vi "water-archive.vi"(1 "C1NI6071E":T1 {"63 ACH63 b100 Libre ?" format="%.3f"; "62 ACH62 b98 Libre ?" format="%.3f"; "61 ACH61 b96 Libre ?" format="%.3f"; "60 ACH60 b94 Libre ?" format="%.3f"; "59 ACH59 b92 Libre ?" format="%.3f"; "58 ACH58 b90 Libre ?" format="%.3f"; "57 ACH57 b88 Libre ?" format="%.3f"; "56 ACH56 b86 Libre ?" format="%.3f"; "55 ACH55 b99 Libre ?" format="%.3f"; "54 ACH54 b97 Libre ?" format="%.3f"; "53 ACH53 b95 Libre ?" format="%.3f"; "52 ACH52 b93 Libre ?" format="%.3f"; "51 ACH51 b91 Libre ?" format="%.3f"; "50 ACH50 b89 Libre ?" format="%.3f"; "49 ACH49 b87 Libre ?" format="%.3f"; "48 ACH48 b85 Réservé" format="%.3f"; "47 ACH47 b84 Réservé" format="%.3f"; "46 ACH46 b82 Réservé" format="%.3f"; "45 ACH45 b80 Mesure phase HF1" format="%.3f"; "44 ACH44 b78 Mesure Atténuateur" format="%.3f"; "43 ACH43 b74 Réservé" format="%.3f"; "42 ACH42 b72 Mes champ Dipôle 2" format="%.3f"; "41 ACH41 b70 Mes H5" format="%.3f"; "40 ACH40 b68 Mes I correcte Dipôle 21 (H4)" format="%.3f"; "39 ACH39 b83 Réservé" format="%.3f"; "38 ACH38 b81 Mesure phase HF2" format="%.3f"; "37 ACH37 b79 Mes position Déphaseur ajust" format="%.3f"; "36 ACH36 b77 Mes position Déphaseur" format="%.3f"; "35 ACH35 b73 Mes champ Dipôle 2" format="%.3f"; "34 ACH34 b71 Mes I Guidage V5" format="%.3f"; "33 ACH33 b69 Mes I Guidage V4" format="%.3f"; "32 ACH32 b67 Mes I Guidage V3" format="%.3f"; "31 ACH31 b66 Mes I correcte Dipôle 1 (H3)" format="%.3f"; "30 ACH30 b64 Mes I Guidage H2" format="%.3f"; "29 ACH29 b62 Mes I Guidage H1" format="%.3f"; "28 ACH28 b60 Mes I Dipôle 1" format="%.3f"; "27 ACH27 b58 Mes I Quadripôle 2" format="%.3f"; "26 ACH26 b56 Réservé" format="%.3f"; "25 ACH25 b54 Mes I Triplet 2-1" format="%.3f"; "24 ACH24 b52 Mes I Triplet 1-2" format="%.3f"; "23 ACH23 b65 Mes I Guidage V2" format="%.3f"; "22 ACH22 b63 Mes I Guidage V1" format="%.3f"; "21 ACH21 b61 Mes I Dipôle 2" format="%.3f"; "20 ACH20 b59 Mes I Solénoïde" format="%.3f"; "19 ACH19 b57 Mes I Quadripôle 1" format="%.3f"; "18 ACH18 b55 Mes I Triplet 2-2" format="%.3f"; "17 ACH17 b53 Réservé" format="%.3f"; "16 ACH16 b51 Mes I Triplet 1-1" format="%.3f"; "15 ACH15 b18 Libre ?" format="%.3f"; "14 ACH14 b16 Libre ?" format="%.3f"; "13 ACH13 b14 Libre ?" format="%.3f"; "12 ACH12 b12 Mes Vide jauge canon" format="%.3f"; "11 ACH11 b10 Mes Vide DIP 1 (PIQ27 + 33)" format="%.3f"; "10 ACH10 b08 Mes Vide Section (PIQ 16)" format="%.3f"; "09 ACH09 b06 Mes Vide SAS guide HF" format="%.3f"; "08 ACH08 b04 Mes température Section" format="%.3f"; "07 ACH07 b17 Libre ?" format="%.3f"; "06 ACH06 b15 Libre ?" format="%.3f"; "05 ACH05 b13 Libre ?" format="%.3f"; "04 ACH04 b11 Mes Vide Ecran 1 (PIQ 53-63)" format="%.3f"; "03 ACH03 b09 Mes Vide Miroir (PIQ 21)" format="%.3f"; "02 ACH02 b07 Mes Vide Canon (PIQ 12)" format="%.3f"; "01 ACH01 b05 Mes Vide Chambre de préparation" format="%.3f"; "00 ACH00 b03 Mes température Canon" format="%.3f"}, 2 "archive in":T2={"sync"={"elyse/sync/NI6071E/delay"=1.5500000000000005, "elyse/sync/NI6071E/width"=1.0, "elyse/sync/frequency/delay"=10.0, "elyse/sync/frequency/width"=181000.0, "elyse/sync/WCM/delay"=2177.9, "elyse/sync/WCM/width"=10.0, "elyse/sync/modulator/delay"=2182.400000000002, "elyse/sync/modulator/width"=3.0, "elyse/sync/HF/delay"=2175.0, "elyse/sync/HF/width"=3.0, "elyse/sync/Faraday/delay"=5080.0, "elyse/sync/Faraday/width"=100.0, "elyse/sync/Oscilloscope/delay"=2175.0, "elyse/sync/Oscilloscope/width"=2.8, "elyse/sync/50Hz_20MHz/delay"=1.0, "elyse/sync/50Hz_20MHz/width"=5000.0, "elyse/sync/laser_HF/delay"=0.35, "elyse/sync/laser_HF/width"=0.35, "elyse/sync/IMAC/delay"=2176.0, "elyse/sync/IMAC/width"=100.0, "elyse/sync/laser/delay"=2008.3, "elyse/sync/laser/width"=10.0, "elyse/sync/oscilloscope1/delay"=2175.0, "elyse/sync/oscilloscope1/width"=10.0, "elyse/sync/oscilloscope2/delay"=2175.0, "elyse/sync/oscilloscope2/width"=100.0, "elyse/sync/detection1/delay"=500.0, "elyse/sync/detection1/width"=500.0, "elyse/sync/detection1/delay"=0.3, "elyse/sync/detection2/width"=10.0, "elyse/sync/machine/delay"=2175.0, "elyse/sync/machine/width"=100.0, "elyse/sync/n_selection"=4.0}, "HT"={"elyse/HT/voltage/set_value"=6.5, "elyse/HT/voltage/value"=1.5625e-08, "elyse/HT/current/value"=0.0, "elyse/preamplifier/set_value"=1.5625e-08, "elyse/preamplifier/value"=0.0}, "HF"={"elyse/HF/attenuator/value"=-0.01903046052094623, "elyse/HF/dephaser/value"=-18.585806237727724, "elyse/HF/dephaser/value_manuel"=-78.82860725035081, "elyse/HF/canon/value"=0.0, "elyse/HF/section/value"=-18.585806237727724}, "vacuum"={"elyse/vacuum/preparation_chamber/state"=TRUE, "elyse/vacuum/preparation_chamber/measurement"=0.0, "elyse/vacuum/HF/state"=TRUE, "elyse/vacuum/HF/measurement"=0.0, "elyse/vacuum/canon/state"=TRUE, "elyse/vacuum/canon/measurement"=0.0, "elyse/vacuum/section/state"=TRUE, "elyse/vacuum/section/measurement"=0.0, "elyse/vacuum/dipole1/state"=TRUE, "elyse/vacuum/dipole1/measurement"=0.0, "elyse/vacuum/screen1/state"=TRUE, "elyse/vacuum/screen1/measurement"=0.0, "elyse/vacuum/mirror/state"=TRUE, "elyse/vacuum/mirror/measurement"=0.0, "elyse/vacuum/tpg300_section/state"=TRUE, "elyse/vacuum/tpg300_section/measurement"=0.0, "elyse/vacuum/valves/cathode/state"=FALSE, "elyse/vacuum/valves/injection/state"=FALSE}, "modulator"={"elyse/modulator/focale1/current/value"=0.0, "elyse/modulator/focale2/current/value"=0.0, "elyse/modulator/focale3/current/value"=0.0, "elyse/modulator/LAR/voltage/value"=0.0, "elyse/modulator/line_end/current/value"=0.0, "elyse/modulator/thyratron/currents/power/value"=0.0, "elyse/modulator/thyratron_reservoir/current/value"=0.0, "elyse/modulator/paramagnetization/current/value"=0.0, "elyse/modulator/thyratron/voltages/heating/value"=0.0, "elyse/modulator/thyratron/currents/heating/value"=0.0, "elyse/modulator/klystron/currents/power/value"=0.0, "elyse/modulator/klystron/voltages/power/value"=0.0, "elyse/modulator/klystron/currents/heating/value"=0.0, "elyse/modulator/klystron/voltages/heating/value"=0.0}, "cooling"={"elyse/cooling/section/temperature/set_value"=28.0, "elyse/cooling/section/temperature/measurement"=27.96142578125, "elyse/cooling/canon/temperature/set_value"=20.2, "elyse/cooling/canon/temperature/measurement"=26.69921875}, "magnets"={"elyse/magnets/focale/set_value"=0.0, "elyse/magnets/focale/value"=0.0, "elyse/magnets/phase_HF_laser/set_value"=0.0, "elyse/magnets/phase_HF_laser/value"=0.0, "elyse/magnets/dipole1/set_value"=0.0, "elyse/magnets/dipole1/value"=0.0, "elyse/magnets/dipole2/set_value"=0.0, "elyse/magnets/dipole2/value"=0.0, "elyse/magnets/Cor_H1/set_value"=0.0, "elyse/magnets/Cor_H1/value"=0.0, "elyse/magnets/Cor_V1/set_value"=0.0, "elyse/magnets/Cor_V1/value"=0.0, "elyse/magnets/Cor_H2/set_value"=0.0, "elyse/magnets/Cor_H2/value"=0.0, "elyse/magnets/Cor_V2/set_value"=0.0, "elyse/magnets/Cor_V2/value"=0.0, "elyse/magnets/Cor_H3/set_value"=0.0, "elyse/magnets/Cor_H3/value"=0.0, "elyse/magnets/Cor_V3/set_value"=-5.0, "elyse/magnets/Cor_V3/value"=0.0, "elyse/magnets/Cor_H4/set_value"=0.0, "elyse/magnets/Cor_H4/value"=0.0, "elyse/magnets/Cor_V4/set_value"=0.0, "elyse/magnets/Cor_V4/value"=0.0, "elyse/magnets/Cor_H5/set_value"=0.0, "elyse/magnets/Cor_H5/value"=0.0, "elyse/magnets/Cor_V5/set_value"=0.0, "elyse/magnets/Cor_V5/value"=0.0, "elyse/magnets/triplet1-1/set_value"=0.0, "elyse/magnets/triplet1-1/value"=0.0, "elyse/magnets/triplet1-2/set_value"=0.0, "elyse/magnets/triplet1-2/value"=0.0, "elyse/magnets/triplet2-1/set_value"=0.0, "elyse/magnets/triplet2-1/value"=0.0, "elyse/magnets/triplet2-2/set_value"=0.0, "elyse/magnets/triplet2-2/value"=0.0, "elyse/magnets/qudrupole1/set_value"=0.0, "elyse/magnets/qudrupole1/value"=0.0, "elyse/magnets/qudrupole2/set_value"=0.0, "elyse/magnets/qudrupole2/value"=0.0}, "time"={"elyse/timestamp"=0.0}}) -> (0 "archive out":T2={"sync"={"elyse/sync/NI6071E/delay"=1.5500000000000005, "elyse/sync/NI6071E/width"=1.0, "elyse/sync/frequency/delay"=10.0, "elyse/sync/frequency/width"=181000.0, "elyse/sync/WCM/delay"=2177.9, "elyse/sync/WCM/width"=10.0, "elyse/sync/modulator/delay"=2182.400000000002, "elyse/sync/modulator/width"=3.0, "elyse/sync/HF/delay"=2175.0, "elyse/sync/HF/width"=3.0, "elyse/sync/Faraday/delay"=5080.0, "elyse/sync/Faraday/width"=100.0, "elyse/sync/Oscilloscope/delay"=2175.0, "elyse/sync/Oscilloscope/width"=2.8, "elyse/sync/50Hz_20MHz/delay"=1.0, "elyse/sync/50Hz_20MHz/width"=5000.0, "elyse/sync/laser_HF/delay"=0.35, "elyse/sync/laser_HF/width"=0.35, "elyse/sync/IMAC/delay"=2176.0, "elyse/sync/IMAC/width"=100.0, "elyse/sync/laser/delay"=2008.3, "elyse/sync/laser/width"=10.0, "elyse/sync/oscilloscope1/delay"=2175.0, "elyse/sync/oscilloscope1/width"=10.0, "elyse/sync/oscilloscope2/delay"=2175.0, "elyse/sync/oscilloscope2/width"=100.0, "elyse/sync/detection1/delay"=500.0, "elyse/sync/detection1/width"=500.0, "elyse/sync/detection1/delay"=0.3, "elyse/sync/detection2/width"=10.0, "elyse/sync/machine/delay"=2175.0, "elyse/sync/machine/width"=100.0, "elyse/sync/n_selection"=4.0}, "HT"={"elyse/HT/voltage/set_value"=6.5, "elyse/HT/voltage/value"=1.5625e-08, "elyse/HT/current/value"=0.0, "elyse/preamplifier/set_value"=1.5625e-08, "elyse/preamplifier/value"=0.0}, "HF"={"elyse/HF/attenuator/value"=-0.01903046052094623, "elyse/HF/dephaser/value"=-18.585806237727724, "elyse/HF/dephaser/value_manuel"=-78.82860725035081, "elyse/HF/canon/value"=0.0, "elyse/HF/section/value"=-18.585806237727724}, "vacuum"={"elyse/vacuum/preparation_chamber/state"=TRUE, "elyse/vacuum/preparation_chamber/measurement"=0.0, "elyse/vacuum/HF/state"=TRUE, "elyse/vacuum/HF/measurement"=0.0, "elyse/vacuum/canon/state"=TRUE, "elyse/vacuum/canon/measurement"=0.0, "elyse/vacuum/section/state"=TRUE, "elyse/vacuum/section/measurement"=0.0, "elyse/vacuum/dipole1/state"=TRUE, "elyse/vacuum/dipole1/measurement"=0.0, "elyse/vacuum/screen1/state"=TRUE, "elyse/vacuum/screen1/measurement"=0.0, "elyse/vacuum/mirror/state"=TRUE, "elyse/vacuum/mirror/measurement"=0.0, "elyse/vacuum/tpg300_section/state"=TRUE, "elyse/vacuum/tpg300_section/measurement"=0.0, "elyse/vacuum/valves/cathode/state"=FALSE, "elyse/vacuum/valves/injection/state"=FALSE}, "modulator"={"elyse/modulator/focale1/current/value"=0.0, "elyse/modulator/focale2/current/value"=0.0, "elyse/modulator/focale3/current/value"=0.0, "elyse/modulator/LAR/voltage/value"=0.0, "elyse/modulator/line_end/current/value"=0.0, "elyse/modulator/thyratron/currents/power/value"=0.0, "elyse/modulator/thyratron_reservoir/current/value"=0.0, "elyse/modulator/paramagnetization/current/value"=0.0, "elyse/modulator/thyratron/voltages/heating/value"=0.0, "elyse/modulator/thyratron/currents/heating/value"=0.0, "elyse/modulator/klystron/currents/power/value"=0.0, "elyse/modulator/klystron/voltages/power/value"=0.0, "elyse/modulator/klystron/currents/heating/value"=0.0, "elyse/modulator/klystron/voltages/heating/value"=0.0}, "cooling"={"elyse/cooling/section/temperature/set_value"=28.0, "elyse/cooling/section/temperature/measurement"=27.96142578125, "elyse/cooling/canon/temperature/set_value"=20.2, "elyse/cooling/canon/temperature/measurement"=26.69921875}, "magnets"={"elyse/magnets/focale/set_value"=0.0, "elyse/magnets/focale/value"=0.0, "elyse/magnets/phase_HF_laser/set_value"=0.0, "elyse/magnets/phase_HF_laser/value"=0.0, "elyse/magnets/dipole1/set_value"=0.0, "elyse/magnets/dipole1/value"=0.0, "elyse/magnets/dipole2/set_value"=0.0, "elyse/magnets/dipole2/value"=0.0, "elyse/magnets/Cor_H1/set_value"=0.0, "elyse/magnets/Cor_H1/value"=0.0, "elyse/magnets/Cor_V1/set_value"=0.0, "elyse/magnets/Cor_V1/value"=0.0, "elyse/magnets/Cor_H2/set_value"=0.0, "elyse/magnets/Cor_H2/value"=0.0, "elyse/magnets/Cor_V2/set_value"=0.0, "elyse/magnets/Cor_V2/value"=0.0, "elyse/magnets/Cor_H3/set_value"=0.0, "elyse/magnets/Cor_H3/value"=0.0, "elyse/magnets/Cor_V3/set_value"=-5.0, "elyse/magnets/Cor_V3/value"=0.0, "elyse/magnets/Cor_H4/set_value"=0.0, "elyse/magnets/Cor_H4/value"=0.0, "elyse/magnets/Cor_V4/set_value"=0.0, "elyse/magnets/Cor_V4/value"=0.0, "elyse/magnets/Cor_H5/set_value"=0.0, "elyse/magnets/Cor_H5/value"=0.0, "elyse/magnets/Cor_V5/set_value"=0.0, "elyse/magnets/Cor_V5/value"=0.0, "elyse/magnets/triplet1-1/set_value"=0.0, "elyse/magnets/triplet1-1/value"=0.0, "elyse/magnets/triplet1-2/set_value"=0.0, "elyse/magnets/triplet1-2/value"=0.0, "elyse/magnets/triplet2-1/set_value"=0.0, "elyse/magnets/triplet2-1/value"=0.0, "elyse/magnets/triplet2-2/set_value"=0.0, "elyse/magnets/triplet2-2/value"=0.0, "elyse/magnets/qudrupole1/set_value"=0.0, "elyse/magnets/qudrupole1/value"=0.0, "elyse/magnets/qudrupole2/set_value"=0.0, "elyse/magnets/qudrupole2/value"=0.0}, "time"={"elyse/timestamp"=0.0}})   [LabVIEW 2020]
uses:
  archive.ctl
  sync_type_def.ctl
  HT_type-def.ctl
  HF_type_def.ctl
  vacuum_type_def.ctl
  modulator_type_def.ctl
  water_cooling_type_def.ctl
  all_magnets_type_def.ctl
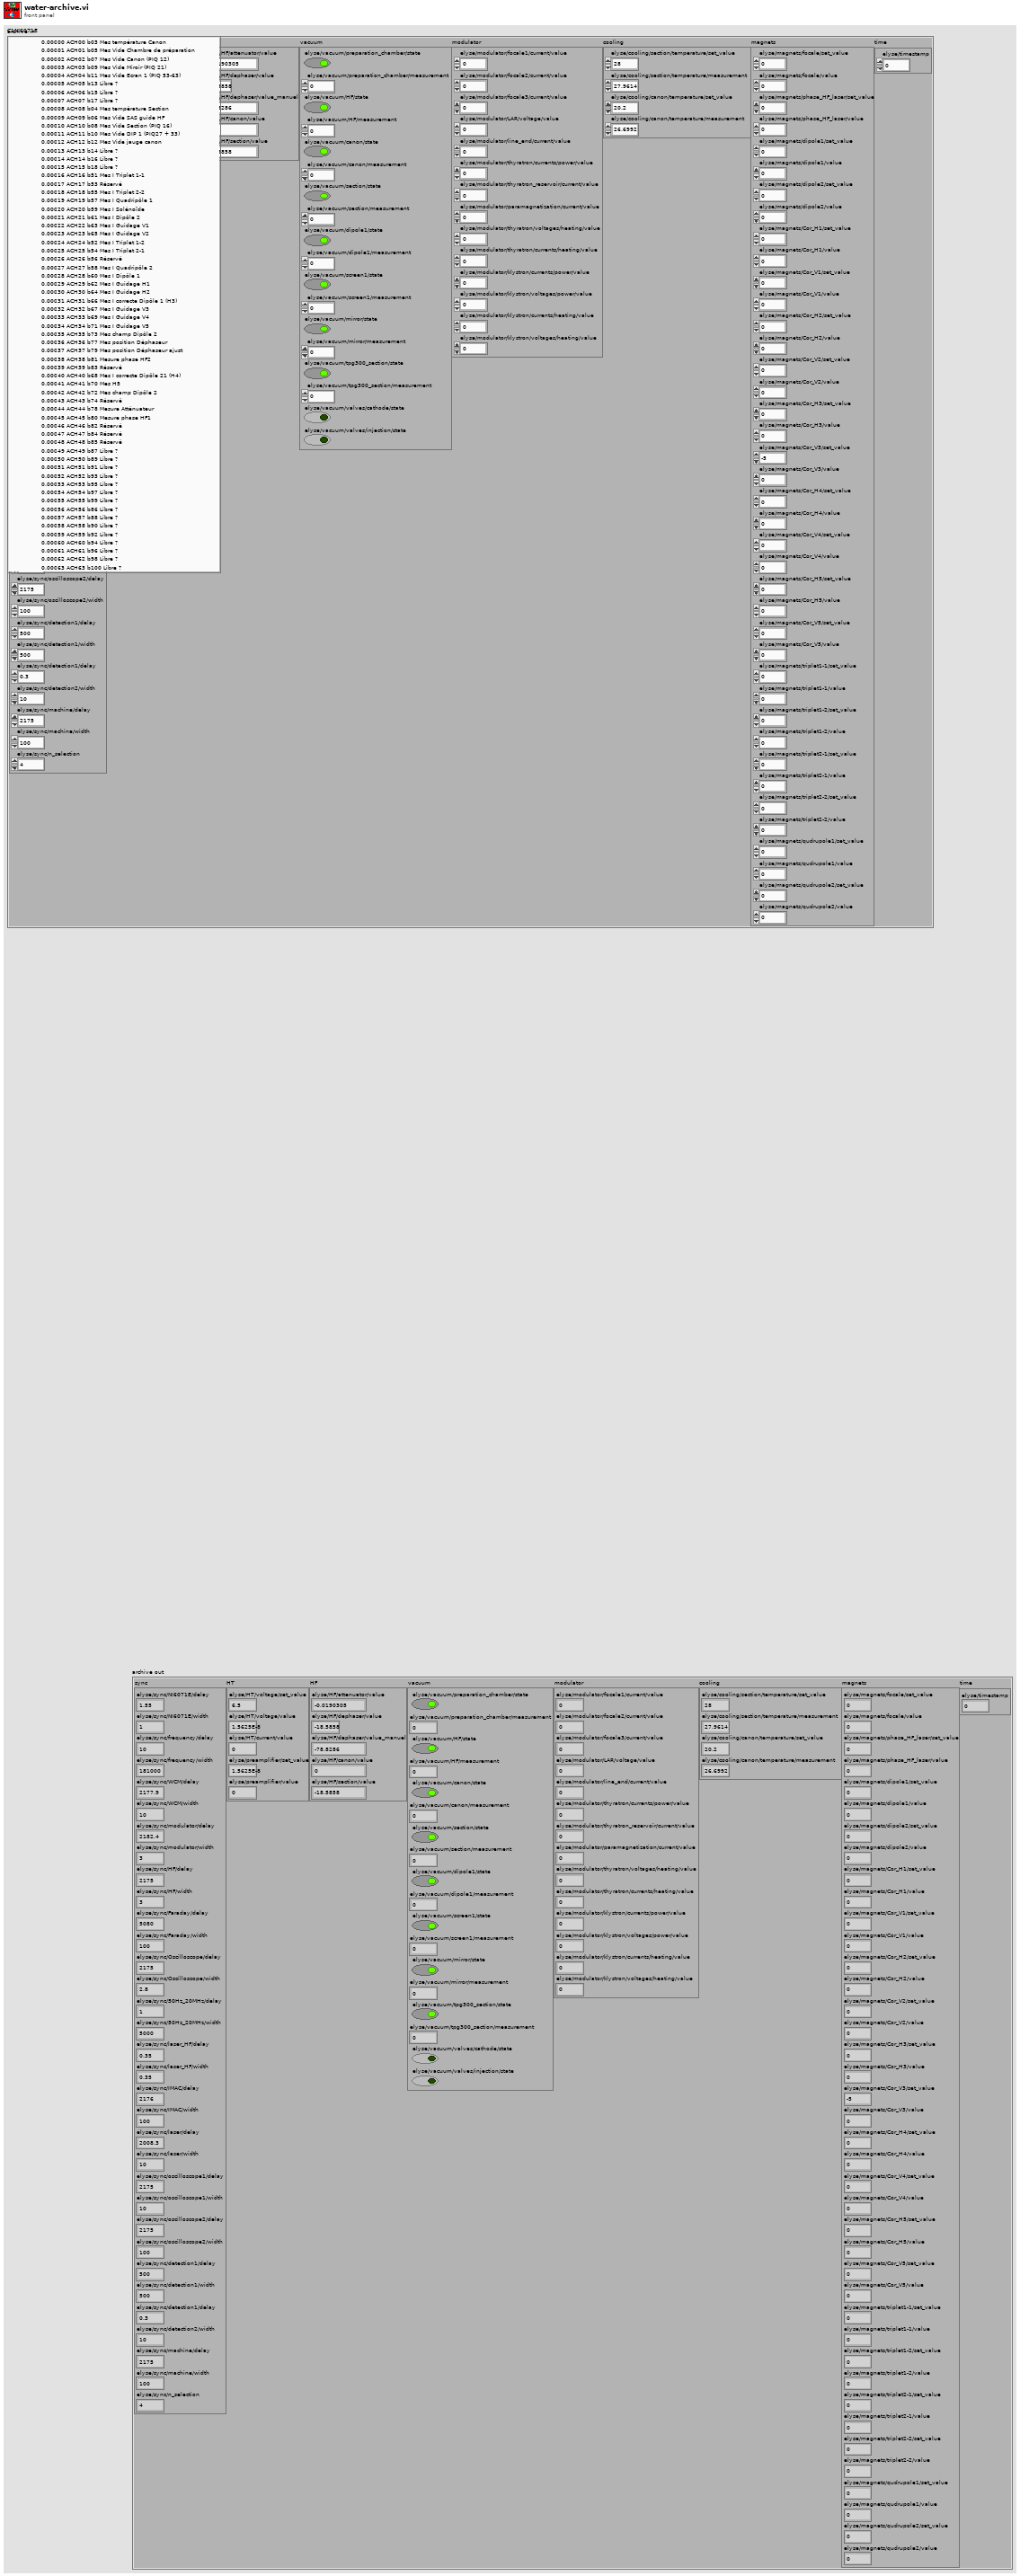
[diagram p1: front panel]
types:
  T1 = cluster{"00 ACH00 b03 Mes température Canon":dbl, "01 ACH01 b05 Mes Vide Chambre de préparation":dbl, "02 ACH02 b07 Mes Vide Canon (PIQ 12)":dbl, "03 ACH03 b09 Mes Vide Miroir (PIQ 21)":dbl, "04 ACH04 b11 Mes Vide Ecran 1 (PIQ 53-63)":dbl, "05 ACH05 b13 Libre ?":dbl, "06 ACH06 b15 Libre ?":dbl, "07 ACH07 b17 Libre ?":dbl, "08 ACH08 b04 Mes température Section":dbl, "09 ACH09 b06 Mes Vide SAS guide HF":dbl, "10 ACH10 b08 Mes Vide Section (PIQ 16)":dbl, "11 ACH11 b10 Mes Vide DIP 1 (PIQ27 + 33)":dbl, "12 ACH12 b12 Mes Vide jauge canon":dbl, "13 ACH13 b14 Libre ?":dbl, "14 ACH14 b16 Libre ?":dbl, "15 ACH15 b18 Libre ?":dbl, "16 ACH16 b51 Mes I Triplet 1-1":dbl, "17 ACH17 b53 Réservé":dbl, "18 ACH18 b55 Mes I Triplet 2-2":dbl, "19 ACH19 b57 Mes I Quadripôle 1":dbl, "20 ACH20 b59 Mes I Solénoïde":dbl, "21 ACH21 b61 Mes I Dipôle 2":dbl, "22 ACH22 b63 Mes I Guidage V1":dbl, "23 ACH23 b65 Mes I Guidage V2":dbl, "24 ACH24 b52 Mes I Triplet 1-2":dbl, "25 ACH25 b54 Mes I Triplet 2-1":dbl, "26 ACH26 b56 Réservé":dbl, "27 ACH27 b58 Mes I Quadripôle 2":dbl, "28 ACH28 b60 Mes I Dipôle 1":dbl, "29 ACH29 b62 Mes I Guidage H1":dbl, "30 ACH30 b64 Mes I Guidage H2":dbl, "31 ACH31 b66 Mes I correcte Dipôle 1 (H3)":dbl, "32 ACH32 b67 Mes I Guidage V3":dbl, "33 ACH33 b69 Mes I Guidage V4":dbl, "34 ACH34 b71 Mes I Guidage V5":dbl, "35 ACH35 b73 Mes champ Dipôle 2":dbl, "36 ACH36 b77 Mes position Déphaseur":dbl, "37 ACH37 b79 Mes position Déphaseur ajust":dbl, "38 ACH38 b81 Mesure phase HF2":dbl, "39 ACH39 b83 Réservé":dbl, "40 ACH40 b68 Mes I correcte Dipôle 21 (H4)":dbl, "41 ACH41 b70 Mes H5":dbl, "42 ACH42 b72 Mes champ Dipôle 2":dbl, "43 ACH43 b74 Réservé":dbl, "44 ACH44 b78 Mesure Atténuateur":dbl, "45 ACH45 b80 Mesure phase HF1":dbl, "46 ACH46 b82 Réservé":dbl, "47 ACH47 b84 Réservé":dbl, "48 ACH48 b85 Réservé":dbl, "49 ACH49 b87 Libre ?":dbl, "50 ACH50 b89 Libre ?":dbl, "51 ACH51 b91 Libre ?":dbl, "52 ACH52 b93 Libre ?":dbl, "53 ACH53 b95 Libre ?":dbl, "54 ACH54 b97 Libre ?":dbl, "55 ACH55 b99 Libre ?":dbl, "56 ACH56 b86 Libre ?":dbl, "57 ACH57 b88 Libre ?":dbl, "58 ACH58 b90 Libre ?":dbl, "59 ACH59 b92 Libre ?":dbl, "60 ACH60 b94 Libre ?":dbl, "61 ACH61 b96 Libre ?":dbl, "62 ACH62 b98 Libre ?":dbl, "63 ACH63 b100 Libre ?":dbl}
  T2 = typedef "archive.ctl" = cluster{"sync":T3, "HT":T4, "HF":T5, "vacuum":T6, "modulator":T7, "cooling":T8, "magnets":T9, "time":cluster{"elyse/timestamp":dbl}}
  T3 = typedef "sync_type_def.ctl" = cluster{"elyse/sync/NI6071E/delay":dbl, "elyse/sync/NI6071E/width":dbl, "elyse/sync/frequency/delay":dbl, "elyse/sync/frequency/width":dbl, "elyse/sync/WCM/delay":dbl, "elyse/sync/WCM/width":dbl, "elyse/sync/modulator/delay":dbl, "elyse/sync/modulator/width":dbl, "elyse/sync/HF/delay":dbl, "elyse/sync/HF/width":dbl, "elyse/sync/Faraday/delay":dbl, "elyse/sync/Faraday/width":dbl, "elyse/sync/Oscilloscope/delay":dbl, "elyse/sync/Oscilloscope/width":dbl, "elyse/sync/50Hz_20MHz/delay":dbl, "elyse/sync/50Hz_20MHz/width":dbl, "elyse/sync/laser_HF/delay":dbl, "elyse/sync/laser_HF/width":dbl, "elyse/sync/IMAC/delay":dbl, "elyse/sync/IMAC/width":dbl, "elyse/sync/laser/delay":dbl, "elyse/sync/laser/width":dbl, "elyse/sync/oscilloscope1/delay":dbl, "elyse/sync/oscilloscope1/width":dbl, "elyse/sync/oscilloscope2/delay":dbl, "elyse/sync/oscilloscope2/width":dbl, "elyse/sync/detection1/delay":dbl, "elyse/sync/detection1/width":dbl, "elyse/sync/detection1/delay":dbl, "elyse/sync/detection2/width":dbl, "elyse/sync/machine/delay":dbl, "elyse/sync/machine/width":dbl, "elyse/sync/n_selection":dbl}
  T4 = typedef "HT_type-def.ctl" = cluster{"elyse/HT/voltage/set_value":dbl, "elyse/HT/voltage/value":dbl, "elyse/HT/current/value":dbl, "elyse/preamplifier/set_value":dbl, "elyse/preamplifier/value":dbl}
  T5 = typedef "HF_type_def.ctl" = cluster{"elyse/HF/attenuator/value":dbl, "elyse/HF/dephaser/value":dbl, "elyse/HF/dephaser/value_manuel":dbl, "elyse/HF/canon/value":dbl, "elyse/HF/section/value":dbl}
  T6 = typedef "vacuum_type_def.ctl" = cluster{"elyse/vacuum/preparation_chamber/state":bool, "elyse/vacuum/preparation_chamber/measurement":dbl, "elyse/vacuum/HF/state":bool, "elyse/vacuum/HF/measurement":dbl, "elyse/vacuum/canon/state":bool, "elyse/vacuum/canon/measurement":dbl, "elyse/vacuum/section/state":bool, "elyse/vacuum/section/measurement":dbl, "elyse/vacuum/dipole1/state":bool, "elyse/vacuum/dipole1/measurement":dbl, "elyse/vacuum/screen1/state":bool, "elyse/vacuum/screen1/measurement":dbl, "elyse/vacuum/mirror/state":bool, "elyse/vacuum/mirror/measurement":dbl, "elyse/vacuum/tpg300_section/state":bool, "elyse/vacuum/tpg300_section/measurement":dbl, "elyse/vacuum/valves/cathode/state":bool, "elyse/vacuum/valves/injection/state":bool}
  T7 = typedef "modulator_type_def.ctl" = cluster{"elyse/modulator/focale1/current/value":dbl, "elyse/modulator/focale2/current/value":dbl, "elyse/modulator/focale3/current/value":dbl, "elyse/modulator/LAR/voltage/value":dbl, "elyse/modulator/line_end/current/value":dbl, "elyse/modulator/thyratron/currents/power/value":dbl, "elyse/modulator/thyratron_reservoir/current/value":dbl, "elyse/modulator/paramagnetization/current/value":dbl, "elyse/modulator/thyratron/voltages/heating/value":dbl, "elyse/modulator/thyratron/currents/heating/value":dbl, "elyse/modulator/klystron/currents/power/value":dbl, "elyse/modulator/klystron/voltages/power/value":dbl, "elyse/modulator/klystron/currents/heating/value":dbl, "elyse/modulator/klystron/voltages/heating/value":dbl}
  T8 = typedef "water_cooling_type_def.ctl" = cluster{"elyse/cooling/section/temperature/set_value":dbl, "elyse/cooling/section/temperature/measurement":dbl, "elyse/cooling/canon/temperature/set_value":dbl, "elyse/cooling/canon/temperature/measurement":dbl}
  T9 = typedef "all_magnets_type_def.ctl" = cluster{"elyse/magnets/focale/set_value":dbl, "elyse/magnets/focale/value":dbl, "elyse/magnets/phase_HF_laser/set_value":dbl, "elyse/magnets/phase_HF_laser/value":dbl, "elyse/magnets/dipole1/set_value":dbl, "elyse/magnets/dipole1/value":dbl, "elyse/magnets/dipole2/set_value":dbl, "elyse/magnets/dipole2/value":dbl, "elyse/magnets/Cor_H1/set_value":dbl, "elyse/magnets/Cor_H1/value":dbl, "elyse/magnets/Cor_V1/set_value":dbl, "elyse/magnets/Cor_V1/value":dbl, "elyse/magnets/Cor_H2/set_value":dbl, "elyse/magnets/Cor_H2/value":dbl, "elyse/magnets/Cor_V2/set_value":dbl, "elyse/magnets/Cor_V2/value":dbl, "elyse/magnets/Cor_H3/set_value":dbl, "elyse/magnets/Cor_H3/value":dbl, "elyse/magnets/Cor_V3/set_value":dbl, "elyse/magnets/Cor_V3/value":dbl, "elyse/magnets/Cor_H4/set_value":dbl, "elyse/magnets/Cor_H4/value":dbl, "elyse/magnets/Cor_V4/set_value":dbl, "elyse/magnets/Cor_V4/value":dbl, "elyse/magnets/Cor_H5/set_value":dbl, "elyse/magnets/Cor_H5/value":dbl, "elyse/magnets/Cor_V5/set_value":dbl, "elyse/magnets/Cor_V5/value":dbl, "elyse/magnets/triplet1-1/set_value":dbl, "elyse/magnets/triplet1-1/value":dbl, "elyse/magnets/triplet1-2/set_value":dbl, "elyse/magnets/triplet1-2/value":dbl, "elyse/magnets/triplet2-1/set_value":dbl, "elyse/magnets/triplet2-1/value":dbl, "elyse/magnets/triplet2-2/set_value":dbl, "elyse/magnets/triplet2-2/value":dbl, "elyse/magnets/qudrupole1/set_value":dbl, "elyse/magnets/qudrupole1/value":dbl, "elyse/magnets/qudrupole2/set_value":dbl, "elyse/magnets/qudrupole2/value":dbl}
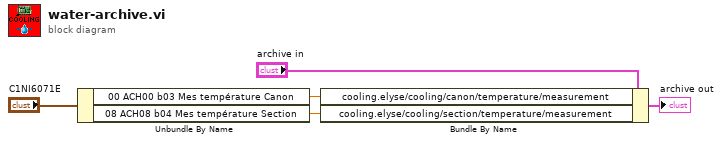
[diagram p0: block diagram]
diagram:
  n1 = Unbundle By Name("C1NI6071E") -> ("00 ACH00 b03 Mes température Canon"=w3:dbl, "08 ACH08 b04 Mes température Section"=w2:dbl)
  n2 = Bundle By Name(cluster="archive in", "cooling.elyse/cooling/canon/temperature/measurement"=w3, "cooling.elyse/cooling/section/temperature/measurement"=w2) -> (→"archive out":T2)
